vi "ReadyCalibFiles.vi"(7 "Cal File Options":T1(ring), 11 "Calib Fnames IN":path[](array[path])) -> (3 "Calib Fnames OUT":path[](array[path]))   [LabVIEW 2015]
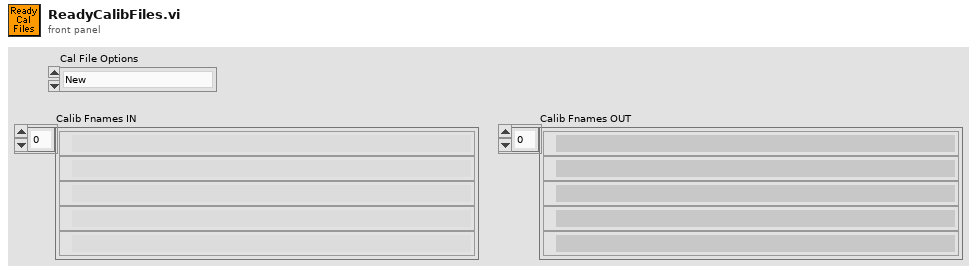
[diagram p1: front panel]
types:
  T1 = enum16{"New", "Add to Current", "Replace Current"}
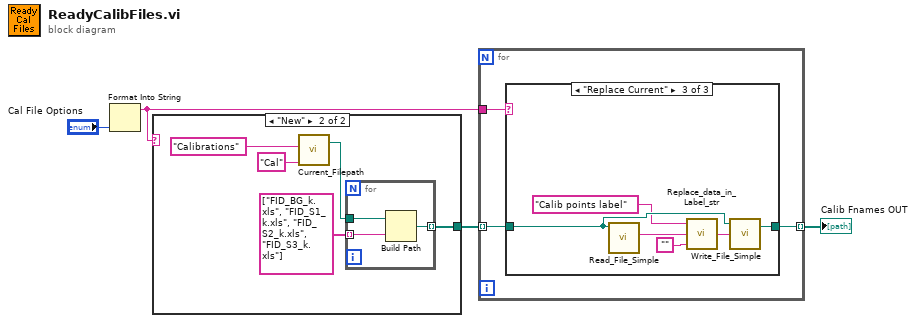
[diagram p0: block diagram]
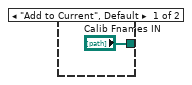
[diagram p2: hidden frame]
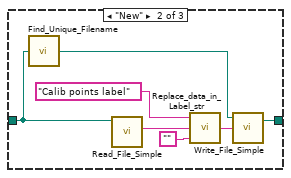
[diagram p4: hidden frame]
diagram:
  n1 = Format Into String("Cal File Options") -> (resulting string=w1:string)  [unwired: 3 in, 1 out]
  n2 = case shown="\"New\"" w1 {
    tunnel: ["Calib Fnames IN" w6] -> w4
    frame "Add to Current", Default {
    }
    frame "New" {
      n3 = call "Current_Filepath.vi"("Short_Name"="Cal" ("Data Type"), "Data Type"="Calibrations") -> ("Directory"=w8:path)  [unwired: 2 in, 1 out]
      n4 = for {
        tunnel: w8 -> [w13]
        tunnel: string[] ["FID_BG_k.xls", "FID_S1_k.xls", "FID_S2_k.xls", "FID_S3_k.xls"] -> [w12] mode=indexing
        tunnel: [w11] -> w6 mode=indexing
        n5 = Build Path(base path=w13, name or relative path=w12) -> (appended path=w11:path)
      }
    }
  }
  n6 = for {
    tunnel: w4 -> [w16] mode=indexing
    tunnel: [w15] -> w3 mode=indexing
    tunnel: w1 -> [w14]
    n7 = case shown="\"Replace Current\"" w14 {
      tunnel: w16 -> [w17 w24 w30]
      tunnel: [w17 w23 w29] -> w15
      frame "Add to Current", Default {
      }
      frame "New" {
        n8 = call "Find_Unique_Filename.vi"("Path In"=w24) -> ("Unique Path Out"=w19:path)  [unwired: 2 in]
        n9 = call "Read_File_Simple.vi"("Filename"=w24) -> ("string"=w21:string)  [unwired: 4 in, 5 out]
        n10 = call "Replace_data_in_Label_str.vi"("New data string"="", "Input string"=w21, "Variable name"="Calib points label") -> ("Appended string"=w18:string)
        n11 = call "Write_File_Simple.vi"("character string"=w18, "file path"=w19) -> ("file path Out"=w23:path)  [unwired: 1 in, 1 out]
      }
      frame "Replace Current" {
        n12 = call "Read_File_Simple.vi"("Filename"=w30) -> ("string"=w27:string)  [unwired: 4 in, 5 out]
        n13 = call "Replace_data_in_Label_str.vi"("New data string"="", "Input string"=w27, "Variable name"="Calib points label") -> ("Appended string"=w25:string)
        n14 = call "Write_File_Simple.vi"("character string"=w25, "file path"=w30) -> ("file path Out"=w29:path)  [unwired: 1 in, 1 out]
      }
    }
  }
  "Calib Fnames OUT" <- w3
